vi "Teleop.vi"(10 "Match Info":T1={"Autonomous Elapsed Seconds"=0.0, "TeleOp Elapsed Seconds"=0.0, "Disabled Elapsed Seconds"=0.0, "Visited Autonomous"=FALSE, "Visited TeleOp"=FALSE, "Visited Disabled"=FALSE, "Autonomous Settings"={"Autonomous Style"=enum."Independent", "VI Refnum"=refnum}}, 11 "Call Context":T2) -> ()   [LabVIEW 2020]
doc: "This VI is called for each enabled TeleOp packet received from the DS. It is typically used to read from joysticks and other inputs and update I/O or setpoints for timed control loops. It should complete and return within 20 milliseconds or risk missing DS packets."
uses:
  <vilib>/Rock Robotics/WPI/DriverStation/WPI_DriverStationDerivedRobotMode.ctl
  <vilib>/Rock Robotics/WPI/DriverStation/WPI_DriverStationMatch Info.ctl
  <vilib>/Rock Robotics/WPI/Utilities/WPI_GetSetVariantRefNum.vi
  <vilib>/Rock Robotics/Network Tables/NT Write Boolean Array.vi
  <vilib>/Rock Robotics/Network Tables/NT Write Numeric Array.vi
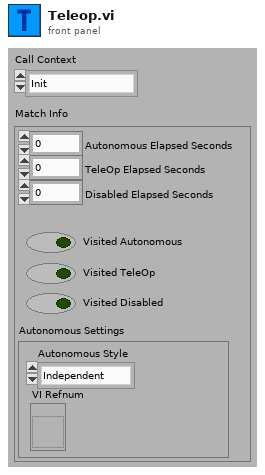
[diagram p1: front panel]
types:
  T1 = typedef "WPI_DriverStationMatch Info.ctl" = cluster{"Autonomous Elapsed Seconds":dbl, "TeleOp Elapsed Seconds":dbl, "Disabled Elapsed Seconds":dbl, "Visited Autonomous":bool, "Visited TeleOp":bool, "Visited Disabled":bool, "Autonomous Settings":cluster{"Autonomous Style":enum16{"Iterative", "Independent"}, "VI Refnum":refnum<vi>}}
  T2 = typedef "WPI_DriverStationDerivedRobotMode.ctl" = enum16{"Init", "Execute", "Stop"}
  T3 = typedef "WPI_JoystickDevRef.ctl" = cluster{"Device":T4}
  T4 = typedef "WPI_JoystickDeviceEnum.ctl" = enum16{"USB 0", "USB 1", "USB 2", "USB 3", "USB 4", "USB 5"}
  T5 = typedef "Command Status Info.ctl" = cluster{"Name":string, "Status":T6, "notifier out":T7}
  T6 = typedef "Completion Status.ctl" = enum16{"Successful", "Aborted", "Incomplete"}
  T7 = typedef "Completion Notifier.ctl" = refnum<notifier>
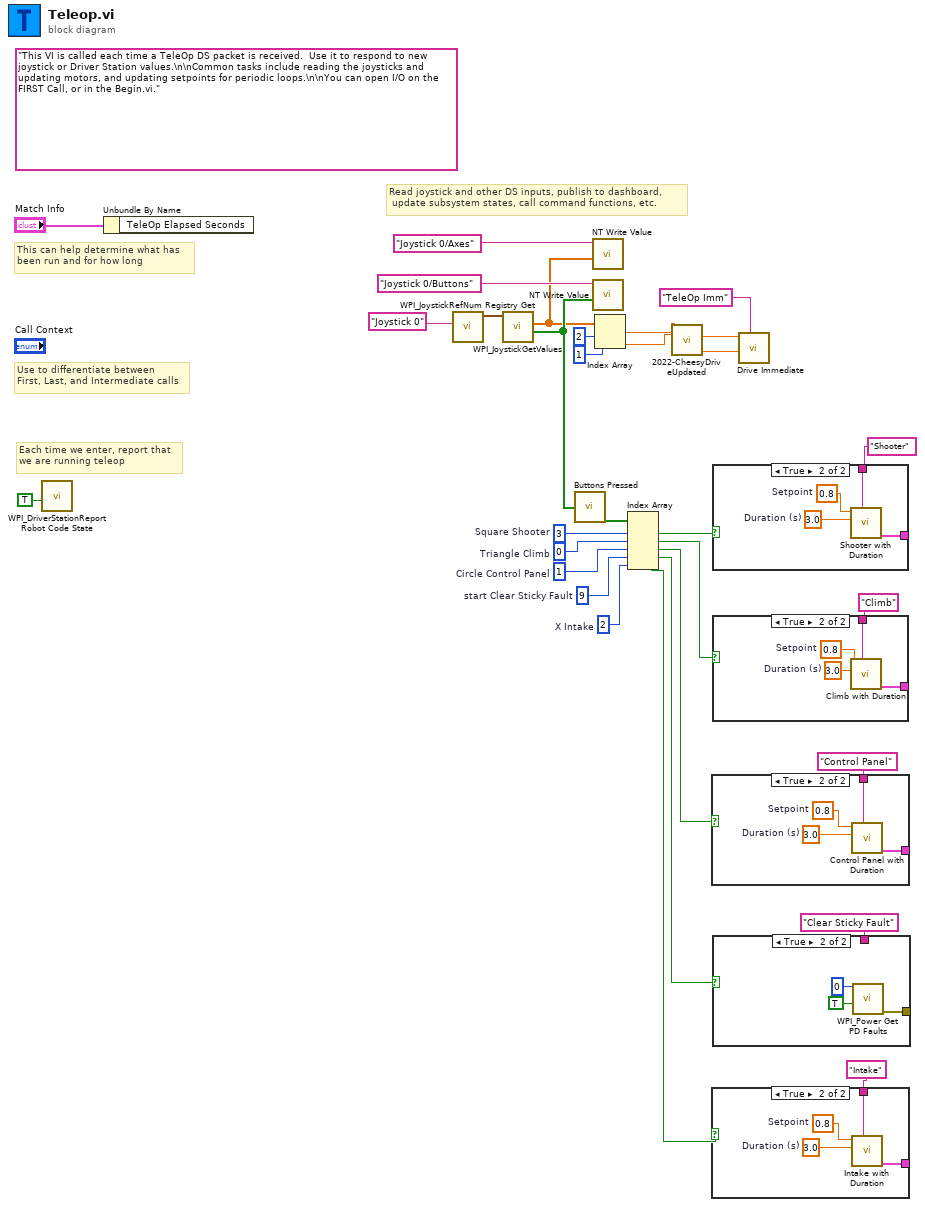
[diagram p0: block diagram]
diagram:
  w5 = 2  # X Intake
  w9 = 9  # start Clear Sticky Fault
  w13 = 1  # Circle Control Panel
  w14 = 0  # Triangle Climb
  w15 = 3  # Square Shooter
  (unwired) "This VI is called each time a TeleOp DS packet is received.  Use it to respond to new joystick or Driver Station values.\n\nCommon tasks include reading the joysticks and updating motors, and updating setpoints for periodic loops.\n\nYou can open I/O on the FIRST Call, or in the Begin.vi."
  # "Read joystick and other DS inputs, publish to dashboard,\n update subsystem states, call command functions, etc."
  # "Each time we enter, report that\nwe are running teleop"
  # "Use to differentiate between\nFirst, Last, and Intermediate calls"
  # "This can help determine what has\nbeen run and for how long"
  n1 = call <vilib>:"WPI_DriverStationReport Robot Code State.vi"("TeleOp"=TRUE ("Autonomous")) -> ()  [unwired: 10 in, 1 out]
  n2 = Unbundle By Name("Match Info") -> ()  [unwired: 1 out]
  n3 = call <vilib>:"WPI_JoystickRefNum Registry Get.vi"("refnum name"="Joystick 0") -> ("JoystickDevRef"=w28:T3)  [unwired: 1 in, 9 out]
  n4 = call <vilib>:"WPI_JoystickGetValues.vi"("JoystickDevRef"=w28) -> ("Buttons"=w18:bool[], "Axes"=w17:dbl[])  [unwired: 6 in, 3 out]
  n5 = call "Buttons Pressed.vi"("Button Values"=w18) -> ("Button Presses"=w24:bool[])
  n6 = call-poly <vilib>:"NT Write Value.vi"("Numeric Array"=w17, "Name"="Joystick 0/Axes") -> ()  [unwired: 9 in, 1 out]
  n7 = call-poly <vilib>:"NT Write Value.vi"("Boolean Array"=w18, "Name"="Joystick 0/Buttons") -> ()  [unwired: 9 in, 1 out]
  n8 = Index Array(array=w17, index #1=2 ("index"), index #2=1 ("index")) -> (element #1=w2:dbl, element #2=w1:dbl)
  n9 = Index Array(array=w24, index #1=w15, index #2=w14, index #3=w13, index #4=w9, index #5=w5) -> (element #1=w23:bool, element #2=w22:bool, element #3=w11:bool, element #4=w8:bool, element #5=w3:bool)
  n10 = call "2022-CheesyDriveUpdated.vi"("Throttle"=w2, "Wheel"=w1) -> ("Left PWM"=w21:dbl, "Right PWM"=w20:dbl)  [unwired: 11 in, 1 out]
  n11 = case shown="True" w11 {
    tunnel: [_ w35] -> _
    tunnel: "Control Panel" ("Description") -> [_ w34]
    frame False {
    }
    frame True {
      w32 = 3.0  # Duration (s)
      w33 = 0.8  # Setpoint
      n12 = call "Control Panel with Duration.vi"("Description"=w34, "Duration (s)"=w32, "Setpoint"=w33) -> ("Command Info Out"=w35:T5)  [unwired: 8 in]
    }
  }
  n13 = case shown="True" w3 {
    tunnel: [_ w39] -> _
    tunnel: "Intake" ("Description") -> [_ w38]
    frame False {
    }
    frame True {
      w36 = 3.0  # Duration (s)
      w37 = 0.8  # Setpoint
      n14 = call "Intake with Duration.vi"("Description"=w38, "Duration (s)"=w36, "Setpoint"=w37) -> ("Command Info Out"=w39:T5)  [unwired: 8 in]
    }
  }
  n15 = case shown="True" w23 {
    tunnel: [_ w43] -> _
    tunnel: "Shooter" ("Description") -> [_ w42]
    frame False {
    }
    frame True {
      w40 = 3.0  # Duration (s)
      w41 = 0.8  # Setpoint
      n16 = call "Shooter with Duration.vi"("Description"=w42, "Duration (s)"=w40, "Setpoint"=w41) -> ("Command Info Out"=w43:T5)  [unwired: 8 in]
    }
  }
  n17 = case shown="True" w22 {
    tunnel: [_ w47] -> _
    tunnel: "Climb" ("Description") -> [_ w46]
    frame False {
    }
    frame True {
      w44 = 0.8  # Setpoint
      w45 = 3.0  # Duration (s)
      n18 = call "Climb with Duration.vi"("Description"=w46, "Duration (s)"=w45, "Setpoint"=w44) -> ("Command Info Out"=w47:T5)  [unwired: 8 in]
    }
  }
  n19 = case shown="True" w8 {
    tunnel: [_ w50] -> _
    tunnel: "Clear Sticky Fault" ("Description") -> [_ _]
    frame False {
    }
    frame True {
      n20 = call <vilib>:"WPI_Power Get PD Faults.vi"("Power Distribution (def)"=u8 0, "Clear Sticky Faults"=TRUE) -> ("error out"=w50:errorcluster)  [unwired: 10 in, 3 out]
    }
  }
  n21 = call "Drive Immediate.vi"("Description"="TeleOp Imm", "Right Setpoint"=w20, "Left Setpoint"=w21) -> ()  [unwired: 8 in, 1 out]
